vi "AIR_QUALITY.vi"() -> ()   [LabVIEW 2019]
uses:
  System.Speech
  <vilib>/numeric/Random Number (Range) I64.vi
panel:
  out "STATEMENT":string
  in  "Iteration   Rate":u32=500
  out "GOOD":bool
  out "MODERATE":bool
  out "WARNING":bool
  in  "?":bool
  out "Air Quality Waveform":i64(graph)
  out "Temperature":i64(slide)=37 scale=0.0..60.0
  out "AIR QUALITY":i64(knob) scale=0.0..300.0
  # "Real Time Air Quality Monitoring"
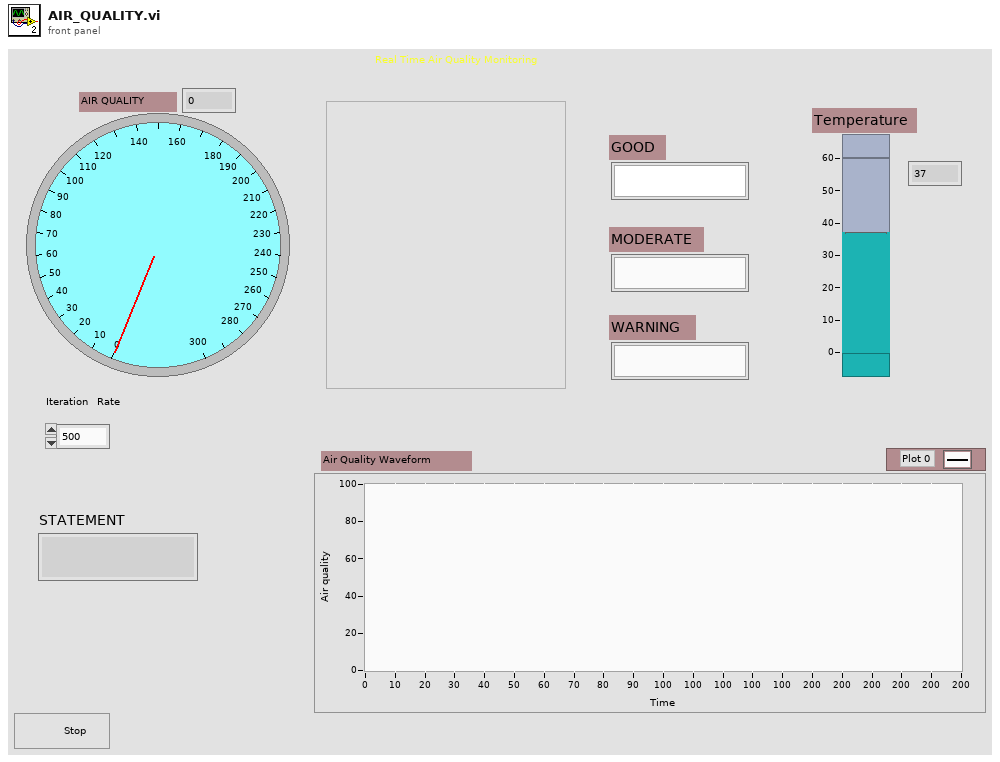
[diagram p1: front panel]
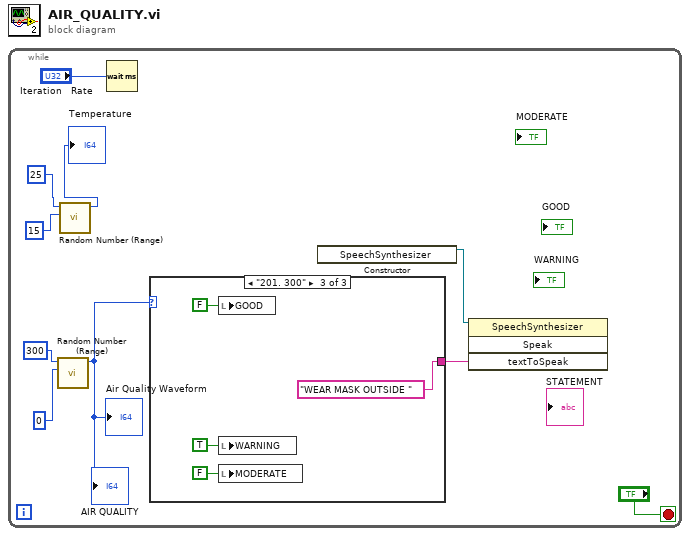
[diagram p0: block diagram]
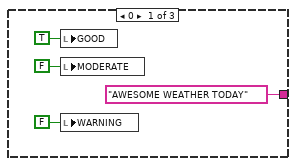
[diagram p2: hidden frame]
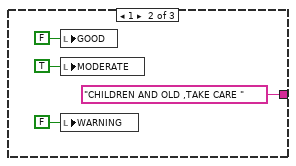
[diagram p3: hidden frame]
diagram:
  n1 = while {
    stop <- "?" stop-if-true
    n2 = call-poly <vilib>:"Random Number (Range).vi"("lower bound (-100)"=u64 0 ("lower bound (0)"), "upper bound (100)"=u64 300) -> ("number"=w1:i64)  [unwired: 9 in]
    "Air Quality Waveform" <- w1
    "AIR QUALITY" <- w1
    n3 = call-poly <vilib>:"Random Number (Range).vi"("lower bound (-100)"=u64 15 ("lower bound (0)"), "upper bound (100)"=u64 25) -> ("number"=→"Temperature":i64)  [unwired: 9 in]
    n4 = Wait (ms)(milliseconds to wait="Iteration   Rate") -> ()  [unwired: 1 out]
    n5 = case shown="\"201. 300\"" w1 {
      tunnel: ["AWESOME WEATHER TODAY" ("textToSpeak") "CHILDREN AND OLD ,TAKE CARE " ("textToSpeak") "WEAR MASK OUTSIDE " ("textToSpeak")] -> w7
      frame 0 {
        n6 = local write "GOOD"(TRUE ("GOOD")) -> ()
        n7 = local write "MODERATE"(FALSE ("GOOD")) -> ()
        n8 = local write "WARNING"(FALSE ("GOOD")) -> ()
      }
      frame 1 {
        n9 = local write "GOOD"(FALSE ("GOOD")) -> ()
        n10 = local write "MODERATE"(TRUE ("GOOD")) -> ()
        n11 = local write "WARNING"(FALSE ("GOOD")) -> ()
      }
      frame 2 {
        n12 = local write "GOOD"(FALSE ("GOOD")) -> ()
        n13 = local write "WARNING"(TRUE ("GOOD")) -> ()
        n14 = local write "MODERATE"(FALSE ("GOOD")) -> ()
      }
    }
    n15 = constructor class="SpeechSynthesizer"() -> (reference out=w8:refnum<k24>)  [unwired: 3 in, 2 out]
    n16 = invoke class="SpeechSynthesizer" method="Speak"(reference=w8, "textToSpeak"=w7) -> ()  [unwired: 2 in, 4 out]
  }
